vi "simpleStatistics.vi"(4 "WiFi Info":T5={"WiFi"={"SSID"="", "Key"=""}, "SystemLink"={"APIKey"="", "Tag"="", "Type"="STRING"}}, 5 "ROI":T2, 6 "Output":enum16{"None", "UART", "SPI", "I2C", "WiFi"}(ring), 7 "Camera Setup":T1={"Format"=enum."RGB565", "size"=enum."QVGA (320x240)", "Skip frames (ms)"=2000, "autoGain"=TRUE, "autoWhitebal"=TRUE}, 8 "error in (no error)":errorcluster, 10 "Statistic":T6(ring), 11 "Python":T3) -> (0 "error out":errorcluster, 2 "Python Code":string, 3 "Python":T3)   [LabVIEW 2024]
uses:
  PythonCtrl.ctl
  Processors.ctl
  _subs/CameraSetup.ctl
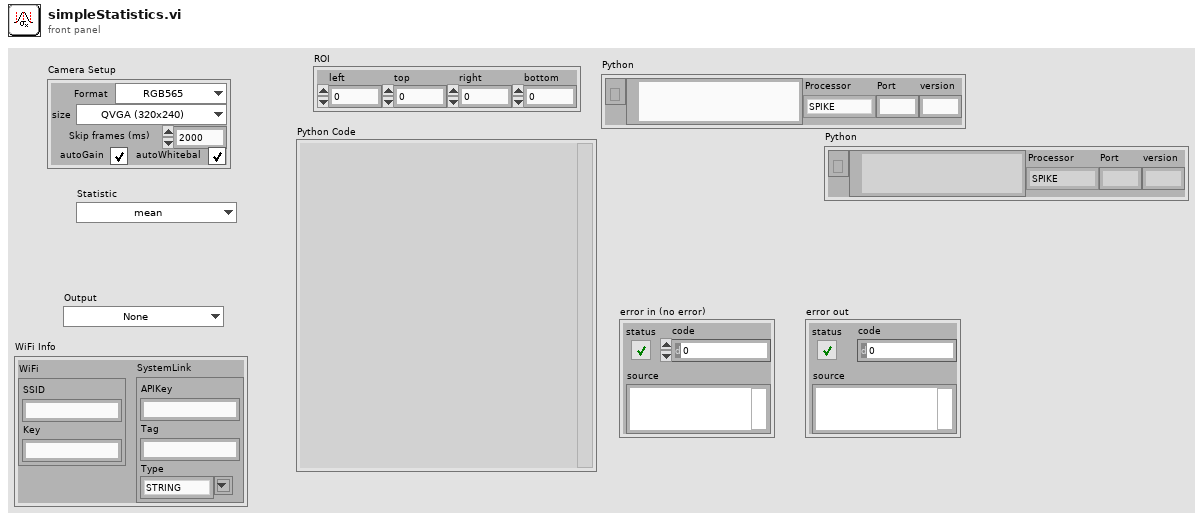
[diagram p1: front panel]
types:
  T1 = typedef "CameraSetup.ctl" = cluster{"Format":enum16{"GRAYSCALE", "RGB565", "BAYER"}, "size":enum16{"QQQQVGA (40x30)", "QQQVGA (80x60)", "QQVGA (160x120)", "QVGA (320x240)", "VGA (640x480)", "LCD (128x160)", "B64x32 (64x32)", "B64x64", "B128x64", "B128x128"}, "Skip frames (ms)":u16, "autoGain":bool, "autoWhitebal":bool}
  T2 = cluster{"left":i32, "top":i32, "right":i32, "bottom":i32}
  T3 = typedef "PythonCtrl.ctl" = cluster{"session":refnum<k35>, "PyPath":path, "Processor":T4, "Port":string, "version":string}
  T4 = typedef "Processors.ctl" = enum16{"SPIKE", "Pi", "Pi_ssh", "OpenMV", "Dunio"}
  T5 = cluster{"WiFi":cluster{"SSID":string, "Key":string}, "SystemLink":cluster{"APIKey":string, "Tag":string, "Type":string}}
  T6 = enum16{"mean", "median", "mode", "sdev", "min", "max", "lower quartile", "upper quartile", "a_mean", "a_median", "a_mode", "a_sdev", "a_min", "a_max", "a_lq", "a_uq", "b_mean", "b_median", "b_mode", "b_sdev", "b_max", "b_min", "b_lq", "b_uq", "All statistics"}
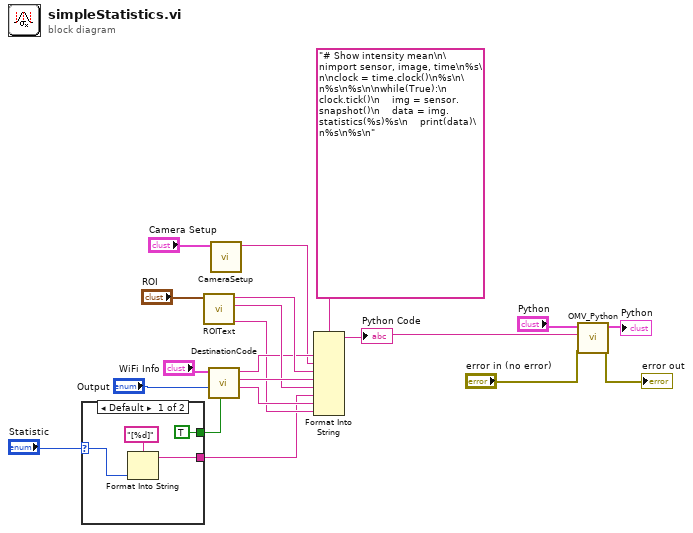
[diagram p0: block diagram]
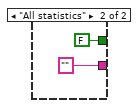
[diagram p2: hidden frame]
diagram:
  n1 = case shown="Default" "Statistic" {
    selector: "Statistic" -> [w23 _]
    tunnel: [w22 ""] -> w5
    tunnel: [TRUE FALSE] -> w4
    frame Default {
      n2 = Format Into String(format string="[%d]", w23) -> (resulting string=w22:string)  [unwired: 2 in, 1 out]
    }
    frame "All statistics" {
    }
  }
  n3 = call "ROIText.vi"("ROI"="ROI") -> ("draw"=w6:string, "roi = r"=w15:string, "r"=w14:string)  [unwired: 7 in, 1 out]
  n4 = call "DestinationCode.vi"("Single number?"=w4, "Destination"="Output", "WiFi Info"="WiFi Info") -> ("Repeated call"=w17:string, "Setup"=w18:string, "Headers"=w13:string)  [unwired: 6 in]
  n5 = call "CameraSetup.vi"("Camera Setup"="Camera Setup") -> ("String"=w12:string)  [unwired: 10 in]
  n6 = Format Into String(format string="# Show intensity mean\n\nimport sensor, image, time\n%s\n\nclock = time.clock()\n%s\n\n%s\n%s\n\nwhile(True):\n    clock.tick()\n    img = sensor.snapshot()\n    data = img.statistics(%s)%s\n    print(data)\n%s\n%s\n" ("startCode"), w13, w12, w14, w18, w15, w5, w17, w6) -> (resulting string=w7:string)  [unwired: 2 in, 1 out]
  "Python Code" <- w7
  n7 = call "OMV_Python.vi"("error in (no error)"="error in (no error)", "Script"=w7, "Python"="Python") -> ("error out"=→"error out":errorcluster, "Python"=→"Python":T3)  [unwired: 7 in]
